vi "OEE_SCREEN_2_recolor_init.vi"(7 "SCREEN_2_recolor_references":T1, 8 "error_in":errorcluster) -> (0 "error_out":errorcluster)   [LabVIEW 2019]
uses:
  typedef/SCREEN_2_recolor_references.ctl
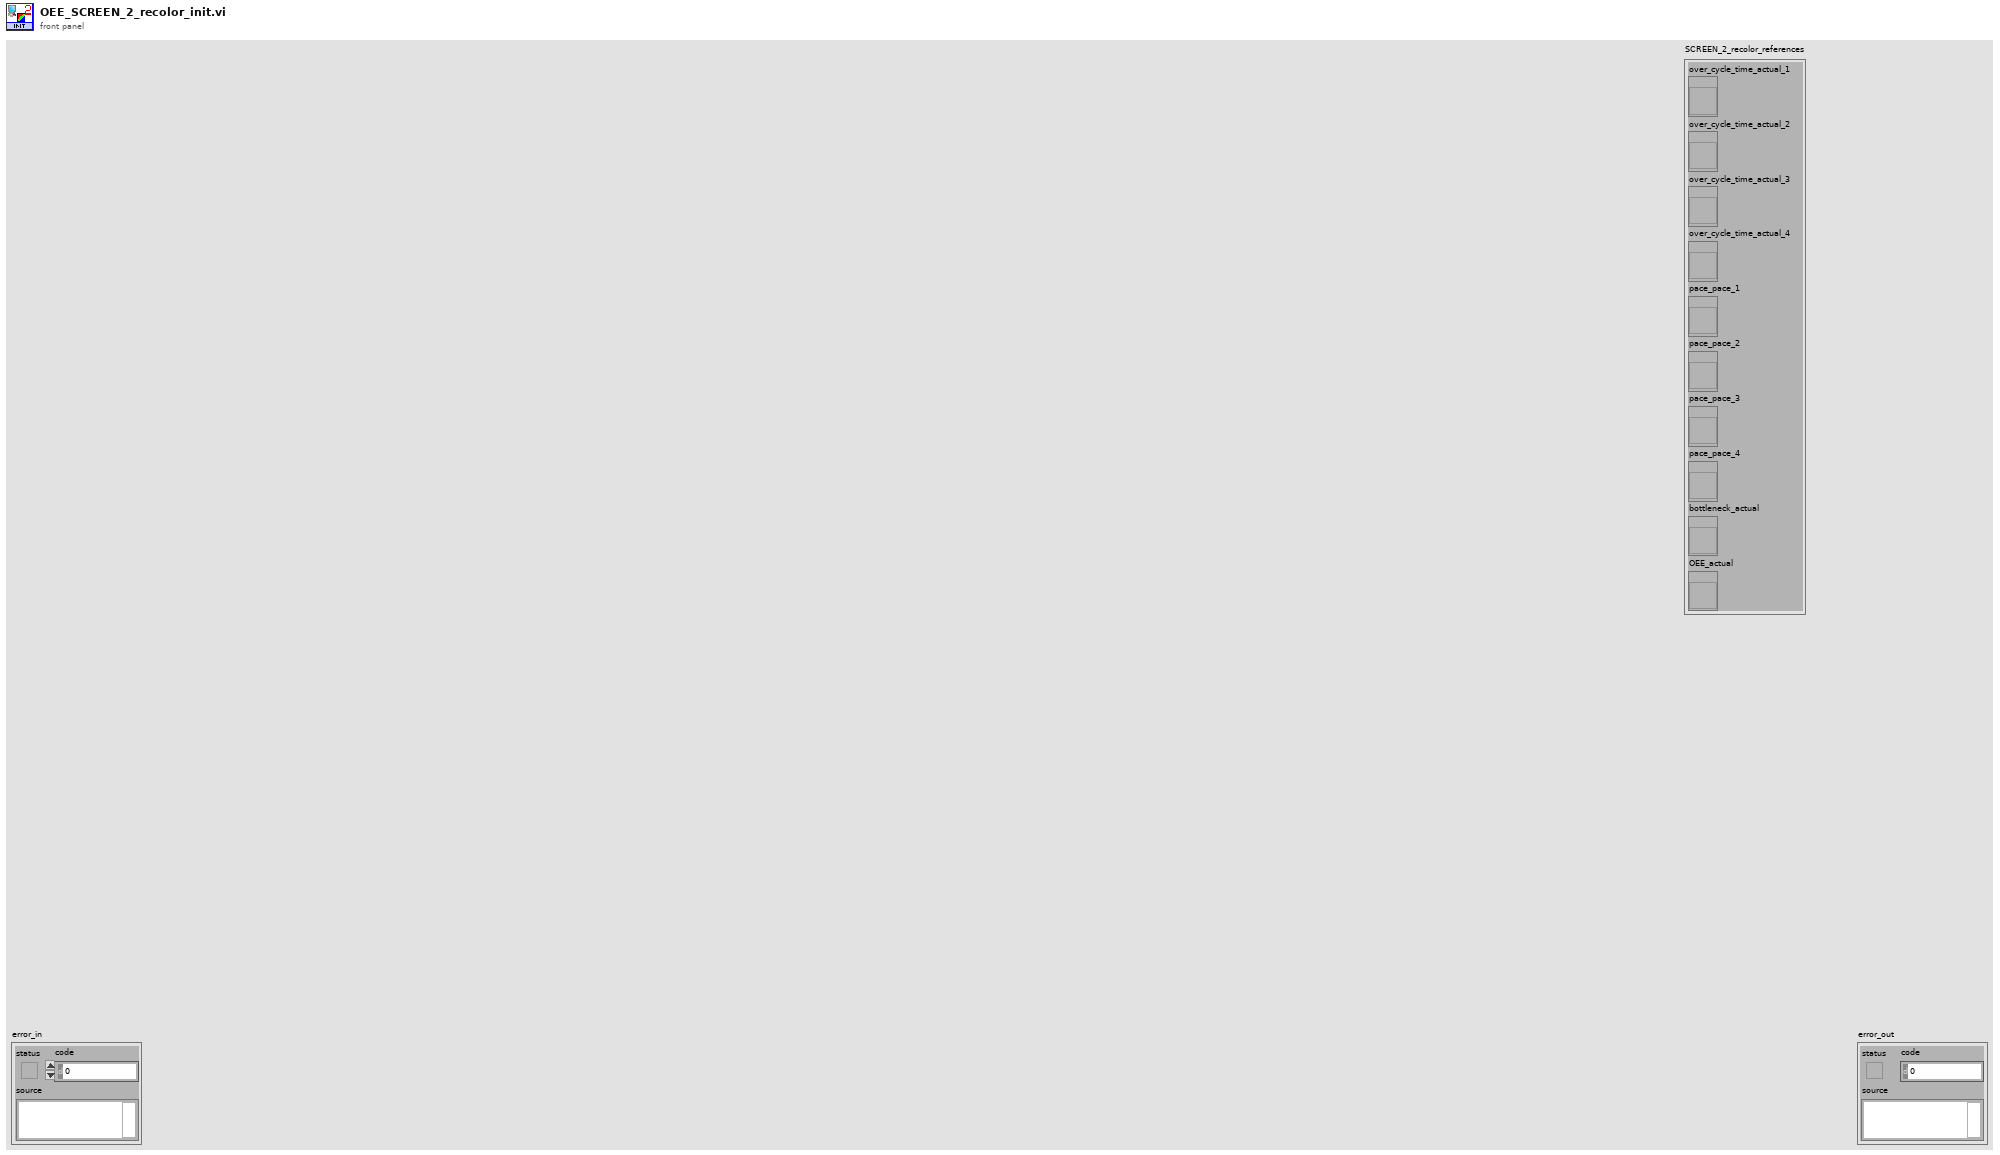
[diagram p1: front panel]
types:
  T1 = typedef "SCREEN_2_recolor_references.ctl" = cluster{"over_cycle_time_actual_1":refnum<vi>, "over_cycle_time_actual_2":refnum<vi>, "over_cycle_time_actual_3":refnum<vi>, "over_cycle_time_actual_4":refnum<vi>, "pace_pace_1":refnum<vi>, "pace_pace_2":refnum<vi>, "pace_pace_3":refnum<vi>, "pace_pace_4":refnum<vi>, "bottleneck_actual":refnum<vi>, "OEE_actual":refnum<vi>}
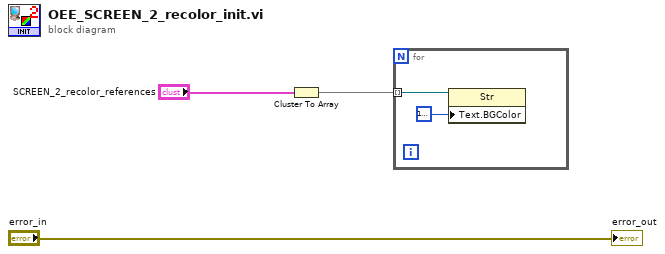
[diagram p0: block diagram]
diagram:
  n1 = Cluster To Array(cluster="SCREEN_2_recolor_references") -> (array=w1:refnum<vi>[])
  n2 = for {
    tunnel: w1 -> [w4] mode=indexing
    n3 = property class="Str"(reference=w4, "Text.BGColor"=u32 16777238) -> ()  [unwired: 1 in, 2 out]
  }
  "error_out" <- "error_in"
